vi "Get Qualified Name.vi"(6 "Path? (F)":bool, 8 "error in (no error)":errorcluster, 11 "SMO":refnum<class "SMO.lvclass">) -> (0 "error out":errorcluster, 2 "Qualified Name":string, 3 "SMO out":refnum<class "SMO.lvclass">)   [LabVIEW 2013, in "SMO.lvclass"]
uses:
  SMO.lvclass
  Support/Attribute.Owner/Attribute.Owner.lvclass
  Support/Attribute.Owner/Attribute.Owner.lvclass/Attribute.Owner.ctl
  Support/Attribute/Attribute.lvclass
panel:
  # "For instructions on how to use the JKI State Machine Objects, examples and video tutorials, visit:\nhttp://jki.net/state-machine-objects/\n\nJKI State Machine Objects™\nhttp://jki.net/state-machine-objects/\nCopyright (C) 2005-2015, JKI <info@jki.net>\nALL RIGHTS RESERVED"
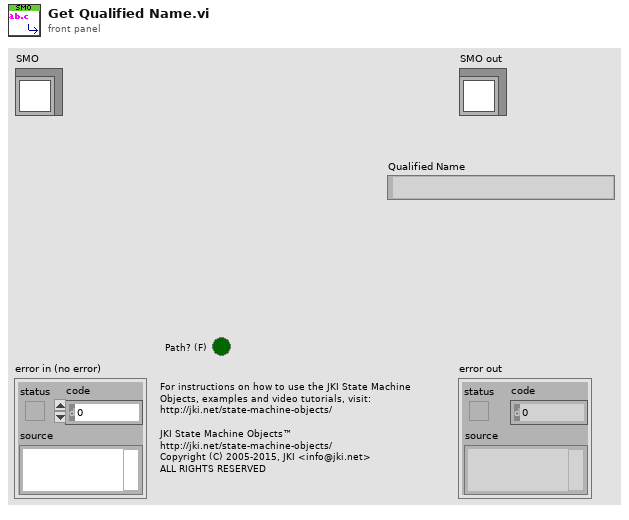
[diagram p1: front panel]
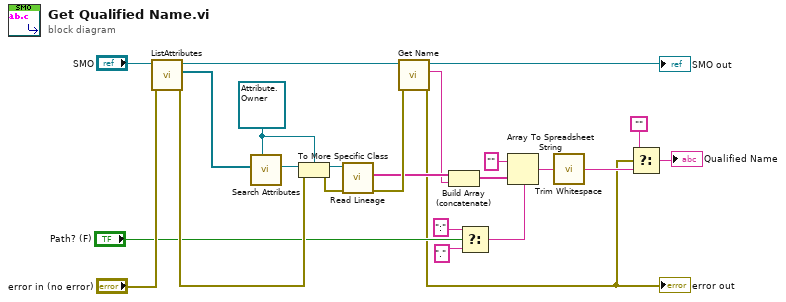
[diagram p0: block diagram]
diagram:
  w18 = refnum<class "Attribute.Owner.lvclass"> refnum ("Attribute.Owner.lvclass")
  n1 = call "ListAttributes.vi"("error in (no error)"="error in (no error)", "SMO in"="SMO") -> ("error out"=w12:errorcluster, "[Attributes]"=w20:refnum<class "Attribute.lvclass">[], "SMO out"=w15:refnum<class "SMO.lvclass">)  [unwired: 7 in]
  n2 = call "Search Attributes.vi"("Attribute type"=w18, "[Attributes]"=w20) -> ("Attribute out"=w24:refnum<class "Attribute.lvclass">)  [unwired: 8 in, 1 out]
  n3 = To More Specific Class(target class=w18, reference=w24, error in=w12) -> (specific class reference=w17:refnum<class "Attribute.Owner.lvclass">, error out=w16:errorcluster)
  n4 = call "Read Lineage.vi"("error in (no error)"=w16, "Attribute.Owner in"=w17) -> ("error out"=w13:errorcluster, "Lineage"=w3:string[])  [unwired: 7 in, 1 out]
  n5 = call "Get Name.vi"("error in (no error)"=w13, "SMO"=w15) -> ("error out"=w1:errorcluster, "Name"=w2:string, "SMO out"=→"SMO out":refnum<class "SMO.lvclass">)  [unwired: 7 in]
  "error out" <- w1
  n6 = Build Array (concatenate)(w3, w2) -> (w11:string[])
  n7 = Select(t=":" ("delimiter (Tab)"), s="Path? (F)", f="." ("delimiter (Tab)")) -> (s? t:f=w4:string)
  n8 = Array To Spreadsheet String(delimiter (Tab)=w4, array=w11, 3:"" ("format string")) -> (spreadsheet string=w9:string)
  n9 = call <vilib>:"Trim Whitespace.vi"("string"=w9) -> ("trimmed string"=w8:string)  [unwired: 1 in]
  n10 = Select(t="", s=w1, f=w8) -> (s? t:f=→"Qualified Name":string)
